vi "BRig_Host_dataqueue_int_array_u16__get.vi"(10 "input_erroDataQueue":errorcluster, 11 "input_hDataQueue":refnum<queue>) -> (0 "output_data":u16[][](array[numeric]), 1 "output_data":bool, 2 "output_errorDataQueue":errorcluster, 3 "output_hDataQueue":refnum<queue>)   [LabVIEW 2014]
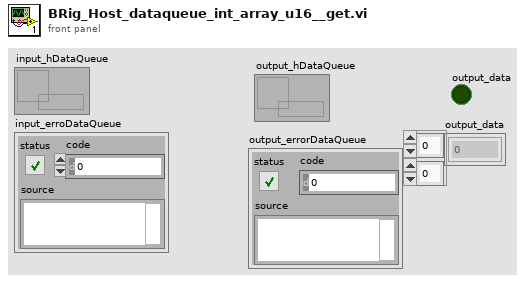
[diagram p1: front panel]
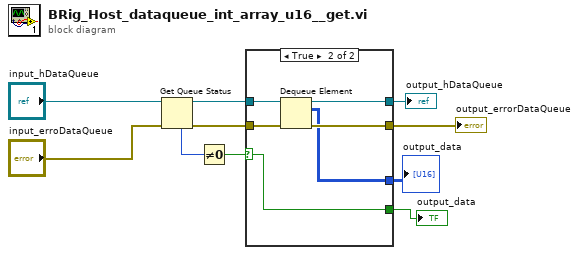
[diagram p0: block diagram]
diagram:
  n1 = Get Queue Status(queue="input_hDataQueue", error in (no error)="input_erroDataQueue") -> (queue out=w3:refnum<queue>, error out=w4:errorcluster, # elements in queue=w8:i32)  [unwired: 1 in, 5 out]
  n2 = Not Equal To 0?(x=w8) -> (x != 0?=w5:bool)
  n3 = case shown="True" w5 {
    selector: w5 -> [w11 w14]
    tunnel: w3 -> [w13 w19]
    tunnel: w4 -> [w12 w18]
    tunnel: [w13 w17] -> w2
    tunnel: [w12 w16] -> w7
    tunnel: [_ w15] -> w1
    tunnel: [w11 w14] -> w6
    frame False {
    }
    frame True {
      n4 = Dequeue Element(queue=w19, error in (no error)=w18) -> (queue out=w17:refnum<queue>, element=w15:u16[][], error out=w16:errorcluster)  [unwired: 1 in, 1 out]
    }
  }
  "output_errorDataQueue" <- w7
  "output_data" <- w6
  "output_hDataQueue" <- w2
  "output_data" <- w1
